vi "calculate binary wppos.vi"(8 "error in (no error)":errorcluster, 11 "S4ICS in":refnum<class "S4ICS.lvclass">) -> (0 "error out":errorcluster, 2 "binary wppos":u32, 3 "S4ICS out":refnum<class "S4ICS.lvclass">)   [LabVIEW 2018]
uses:
  S4ICS.lvclass
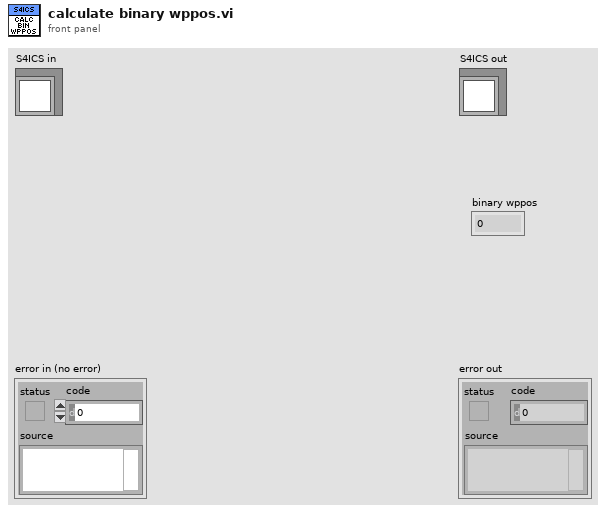
[diagram p1: front panel]
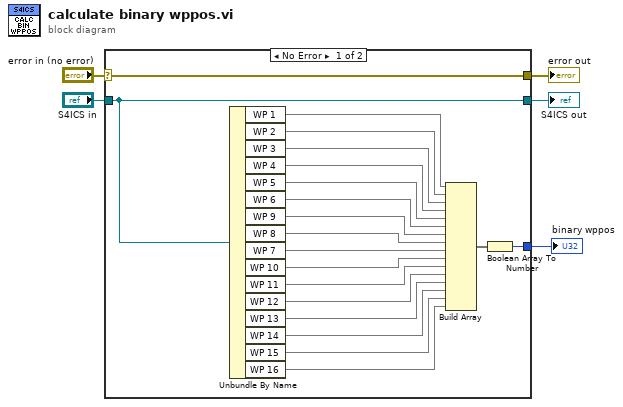
[diagram p0: block diagram]
diagram:
  n1 = case shown="No Error" "error in (no error)" {
    selector: "error in (no error)" -> [w25 w27]
    tunnel: [w25 w27] -> w4
    tunnel: [w24 w26] -> w2
    tunnel: "S4ICS in" -> [w24 w26]
    tunnel: [w6 _] -> w1
    frame No Error {
      n2 = Unbundle By Name(w24) -> ("WP 1"=w23, "WP 2"=w22, "WP 3"=w21, "WP 4"=w20, "WP 5"=w19, "WP 6"=w18, "WP 9"=w17, "WP 8"=w16, "WP 7"=w15, "WP 10"=w14, "WP 11"=w13, "WP 12"=w12, "WP 13"=w11, "WP 14"=w10, "WP 15"=w9, "WP 16"=w8)
      n3 = Build Array(w23, w22, w21, w20, w19, w18, w17, w16, w15, w14, w13, w12, w11, w10, w9, w8) -> (w7:void[])
      n4 = Boolean Array To Number(Boolean array=w7) -> (number=w6:u32)
    }
    frame Error {
    }
  }
  "error out" <- w4
  "S4ICS out" <- w2
  "binary wppos" <- w1
